vi "Visual Analyser.vi"(0 "Image In (RGB overlay)":T1, 1 "Buttons":T2, 2 "Indicators":T7, 3 "Dialog Indicator":refnum<vi>, 4 "Vision Frame":T1, 5 "Image Indicator":variant, 7 "Visualization Parameters":T3, 9 "Image Analysis":T6, 11 "Error In":errorcluster, 12 "Exploration and Autofocus":T4, 13 "Targeting Units":T5(array[cluster]), 14 "Transformation Matrix":refnum<vi>) -> (8 "Vision Frame Out":T1, 15 "Error Out":errorcluster)   [LabVIEW 2012, in "Visual Analyser.lvlib"]
uses:
  Visual Analyser.lvlib
  <vilib>/Analysis/Matrix/Datatypes/RealMatrix.ctl
  <vilib>/vision/Image Controls.llb/IMAQ Image.ctl
  <vilib>/vision/NI_Vision_Development_Module.lvlib
  <vilib>/Analysis/Matrix/NI_Matrix.lvlib
panel:
  out "Image Area":cluster{"X Resolution":i32, "Y Resolution":i32}
  out "Image":T1(plugin-control)
  out "Exit":bool
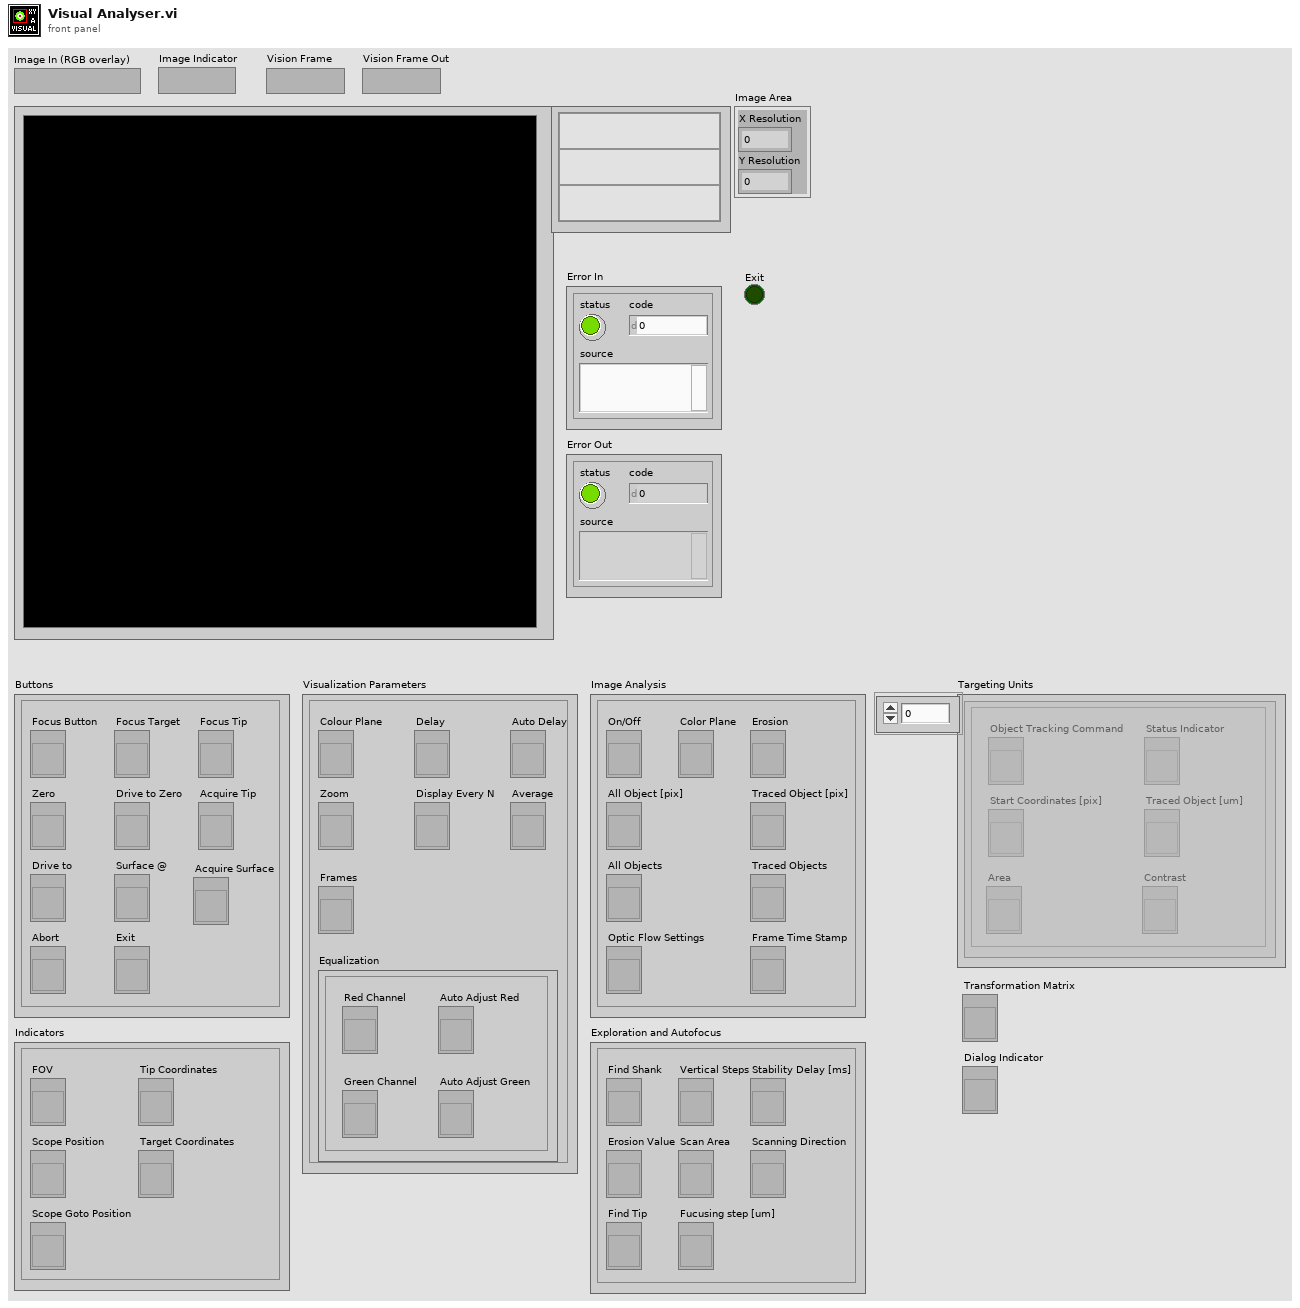
[diagram p1: front panel]
types:
  T1 = typedef "IMAQ Image.ctl" = refnum<image>
  T2 = cluster{"Focus Tip":refnum<vi>, "Focus Target":refnum<vi>, "Drive to Zero":refnum<vi>, "Zero":refnum<vi>, "Acquire Tip":refnum<vi>, "Focus Button":refnum<vi>, "Exit":refnum<vi>, "Abort":refnum<vi>, "Drive to":refnum<vi>, "Surface @":refnum<vi>, "Acquire Surface":refnum<vi>}
  T3 = cluster{"Display Every N":refnum<vi>, "Average":refnum<vi>, "Frames":refnum<vi>, "Colour Plane":refnum<vi>, "Zoom":refnum<vi>, "Delay":refnum<vi>, "Equalization":cluster{"Green Channel":refnum<vi>, "Auto Adjust Green":refnum<vi>, "Red Channel":refnum<vi>, "Auto Adjust Red":refnum<vi>}, "Auto Delay":refnum<vi>}
  T4 = cluster{"Find Shank":refnum<vi>, "Find Tip":refnum<vi>, "Scanning Direction":refnum<vi>, "Scan Area":refnum<vi>, "Stability Delay [ms]":refnum<vi>, "Vertical Steps":refnum<vi>, "Fucusing step [um]":refnum<vi>, "Erosion Value":refnum<vi>}
  T5 = cluster{"Object Tracking Command":refnum<vi>, "Status Indicator":refnum<vi>, "Start Coordinates [pix]":refnum<vi>, "Traced Object [um]":refnum<vi>, "Area":refnum<vi>, "Contrast":refnum<vi>}[]
  T6 = cluster{"On/Off":refnum<vi>, "All Objects":refnum<vi>, "Color Plane":refnum<vi>, "Erosion":refnum<vi>, "Traced Objects":refnum<vi>, "Frame Time Stamp":refnum<vi>, "Optic Flow Settings":refnum<vi>, "All Object [pix]":refnum<vi>, "Traced Object [pix]":refnum<vi>}
  T7 = cluster{"Tip Coordinates":refnum<vi>, "Target Coordinates":refnum<vi>, "Scope Position":refnum<vi>, "FOV":refnum<vi>, "Scope Goto Position":refnum<vi>}
  T8 = cluster{"Area":dbl, "Centre of Mass":cluster{"X":dbl, "Y":dbl}, "Global Rectangle":cluster{"Left":dbl, "Top":dbl, "Right":dbl, "Bottom":dbl}, "Contrast":dbl}[]
  T9 = cluster{"Pyramid Levels":i32, "Max Iterations":i32, "Displacement Threshold":dbl, "Window Size":i32}
  T10 = cluster{"X [um]":dbl, "Y [um]":dbl, "Z [um]":dbl}
  T11 = typedef "NI_Matrix.lvlib/RealMatrix.ctl" = dbl[][]
  T12 = cluster{"Erosion Value":refnum<vi>, "Fucusing step [um]":refnum<vi>, "Stability Delay [ms]":refnum<vi>}
  T13 = cluster{"Vertical Steps":refnum<vi>, "Stability Delay":refnum<vi>, "Scanning Direction":refnum<vi>, "Scan Area":refnum<vi>}
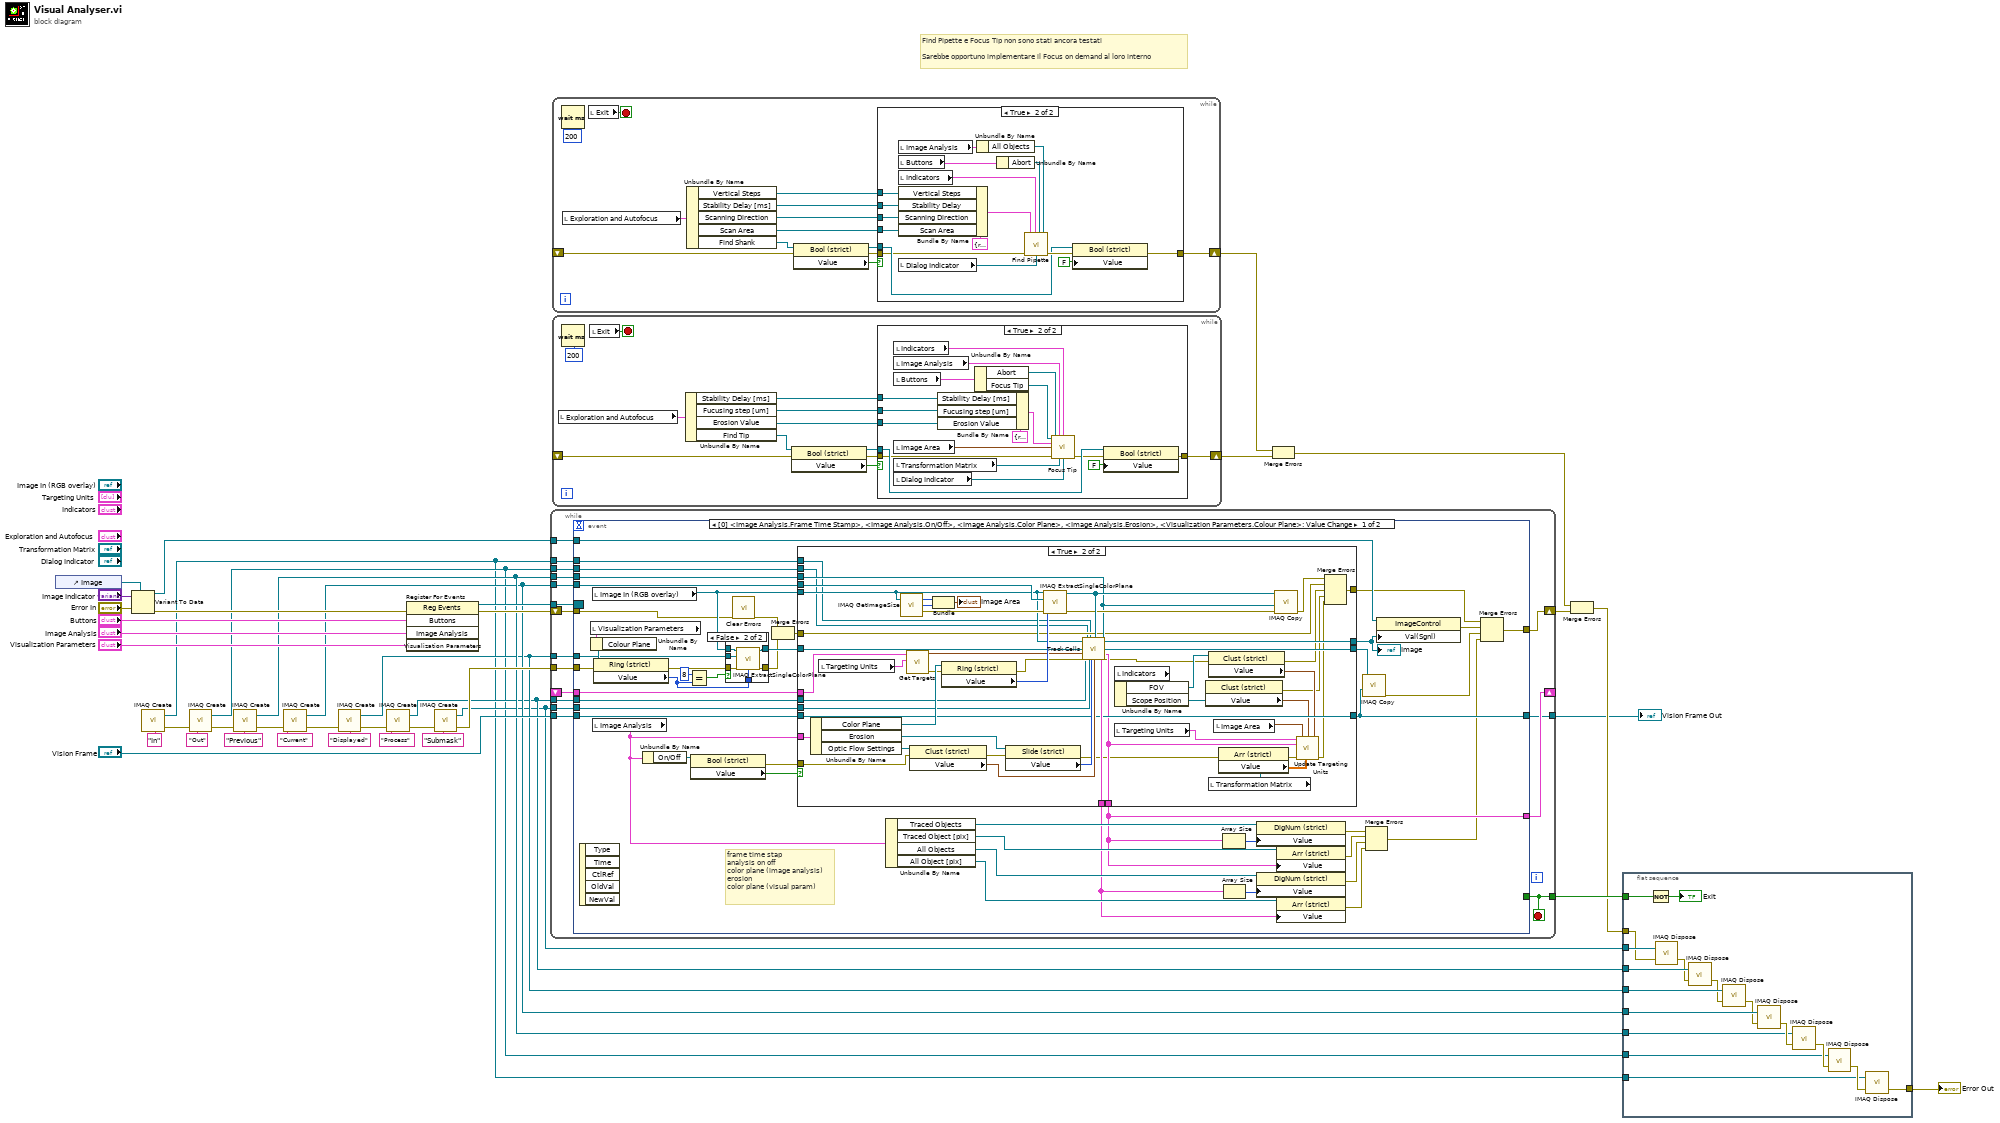
[diagram p0: block diagram]
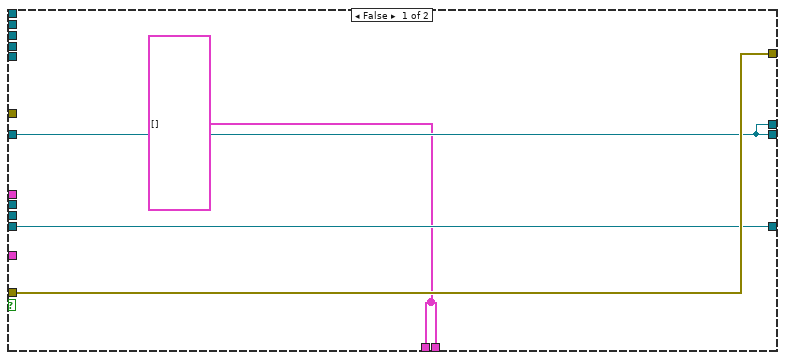
[diagram p5: hidden frame]
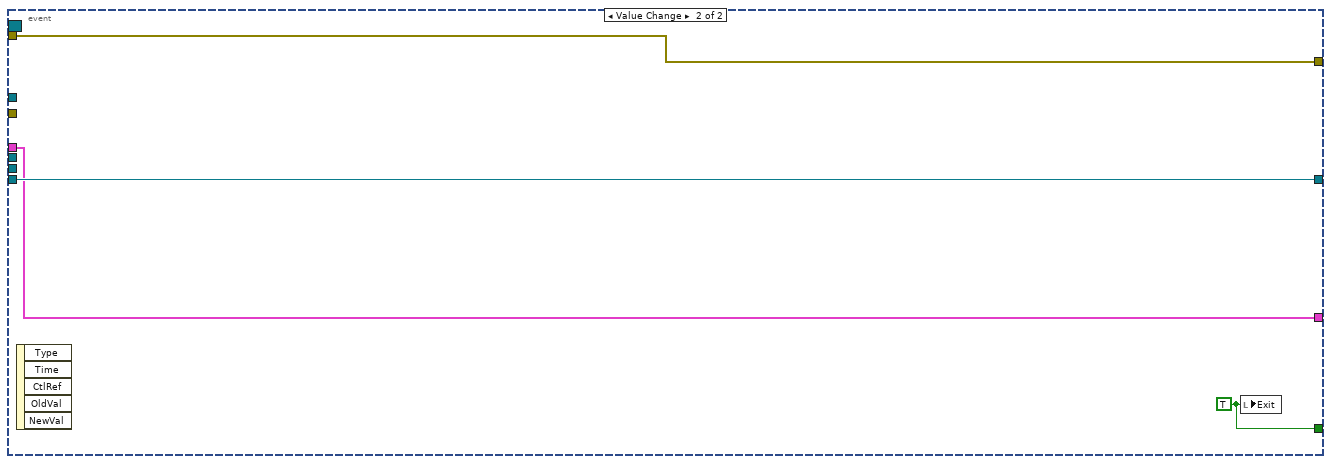
[diagram p6: hidden frame]
diagram:
  # "Find Pipette e Focus Tip non sono stati ancora testati\n\nSarebbe opportuno implementare il Focus on demand al loro interno"
  n1 = control-ref of="Image"() -> (w34:refnum<vi>)
  n2 = Variant To Data(error in="Error In", type=w34, Variant="Image Indicator") -> (data=w36:refnum<vi>, error out=w20:errorcluster)
  n3 = call "IMAQ Create"("Image Name"="In") -> ("New Image"=w1:T1, "error out"=w8:errorcluster)  [unwired: 4 in]
  n4 = call "IMAQ Create"("Image Name"="Out", "error in (no error)"=w8) -> ("New Image"=w2:T1, "error out"=w10:errorcluster)  [unwired: 3 in]
  n5 = call "IMAQ Create"("Image Name"="Previous", "error in (no error)"=w10) -> ("New Image"=w7:T1, "error out"=w32:errorcluster)  [unwired: 3 in]
  n6 = call "IMAQ Create"("Image Name"="Current", "error in (no error)"=w32) -> ("New Image"=w6:T1, "error out"=w24:errorcluster)  [unwired: 3 in]
  n7 = call "IMAQ Create"("Image Name"="Displayed", "error in (no error)"=w24) -> ("New Image"=w5:T1, "error out"=w33:errorcluster)  [unwired: 3 in]
  n8 = call "IMAQ Create"("Image Name"="Process", "error in (no error)"=w33) -> ("New Image"=w4:T1, "error out"=w13:errorcluster)  [unwired: 3 in]
  n9 = register-events(error in=w20, "Buttons", "Image Analysis", "Visualization Parameters") -> (reference out=w22:refnum<event-registration>, error out=w21:errorcluster)  [unwired: 1 in]
  n10 = call "IMAQ Create"("Image Name"="Submask", "error in (no error)"=w13) -> ("New Image"=w3:T1, "error out"=w12:errorcluster)  [unwired: 3 in]
  n11 = while {
    tunnel: w6 -> [w51]
    tunnel: w4 -> [w57]
    tunnel: w5 -> [w56]
    shift-right: [w54] -> _
    shift-left: _ -> [w55]
    tunnel: w36 -> [w49]
    tunnel: [w53] -> w31
    tunnel: w7 -> [w52]
    shift-right: [w47] -> w26
    shift-left: w21 -> [w48]
    tunnel: w12 -> [w50]
    tunnel: w22 -> [w46]
    tunnel: "Vision Frame" -> [w45]
    tunnel: [w44] -> w16
    tunnel: w3 -> [w43]
    tunnel: w2 -> [w42]
    tunnel: w1 -> [w41]
    stop <- w53 stop-if-true
    n12 = event shown="[0] <Image Analysis.Frame Time Stamp>, <Image Analysis.On/Off>, <Image Analysis.Color Plane>, <Image Analysis.Erosion>, <Visualization Parameters.Colour Plane>: Value Change" {
      selector: w46 -> [_ _]
      dyn-events: _ -> [_ _]
      timeout: _ -> [_ _]
      tunnel: w57 -> [w73 _]
      tunnel: w56 -> [w72 _]
      tunnel: w55 -> [w100 w168]
      tunnel: [w79 w168] -> w54
      tunnel: [_ w171] -> w53
      tunnel: w52 -> [w83 _]
      tunnel: w51 -> [w82 _]
      tunnel: w50 -> [w81 _]
      tunnel: w49 -> [w80 _]
      tunnel: w48 -> [w59 w170]
      tunnel: [w60 w170] -> w47
      tunnel: w45 -> [w70 w169]
      tunnel: [w69 w169] -> w44
      tunnel: w43 -> [w67 _]
      tunnel: w42 -> [w66 _]
      tunnel: w41 -> [w65 _]
      event Value Change {
        # "frame time stap\nanalysis on off\ncolor plane (image analysis)\nerosion\ncolor plane (visual param)"
        n13 = event-data() -> ()  [unwired: 1 in, 5 out]
        n14 = local read "Visualization Parameters"() -> (w84:T3)
        n15 = Unbundle By Name(w84) -> ("Colour Plane"=w92:refnum<vi>)
        n16 = local read "Image Analysis"() -> (w78:T6)
        n17 = local read "Image In (RGB overlay)"() -> (w77:T1)
        n18 = property on="Property Node" class="Ring (strict)"(reference=w92, error in=w81) -> (error out=w90:errorcluster, "Value"=w101:i32)  [unwired: 1 out]
        n19 = Unbundle By Name(w78) -> ("On/Off"=w93:refnum<vi>)
        n20 = Equal?(x=8, y=w101) -> (x = y?=w102:bool)
        n21 = property on="Property Node" class="Bool (strict)"(reference=w93) -> (error out=w91:errorcluster, "Value"=w104:bool)  [unwired: 1 in, 1 out]
        n22 = case shown="False" w102 {
          tunnel: w77 -> [w106 w112]
          tunnel: [w106 w111] -> w76
          tunnel: w72 -> [_ w110]
          tunnel: [w105 w109] -> w74
          tunnel: w101 -> [_ w108]
          tunnel: w90 -> [w105 w107]
          frame True {
          }
          frame False {
            n23 = call "IMAQ ExtractSingleColorPlane"("Color Plane"=w108, "error in (no error)"=w107, "Image Dst"=w110, "Image Src"=w112) -> ("error out"=w109:errorcluster, "Image Dst Out"=w111:T1)  [unwired: 6 in]
          }
        }
        n24 = call <vilib>:"Clear Errors.vi"("error in (no error)"=w59) -> ("error out"=w58:errorcluster)  [unwired: 6 in]
        n25 = Merge Errors(w58, w74) -> (w75:errorcluster)
        n26 = case shown="True" w104 {
          tunnel: w83 -> [_ w164]
          tunnel: w73 -> [_ w148]
          tunnel: w76 -> [w114 w149]
          tunnel: w82 -> [_ w155]
          tunnel: w100 -> [_ w143]
          tunnel: [w114 w146] -> w71
          tunnel: w77 -> [_ w125]
          tunnel: w91 -> [w116 w150]
          tunnel: w75 -> [_ w122]
          tunnel: [w116 w151] -> w64
          tunnel: [w113 w161] -> w89
          tunnel: [w113 w144] -> w79
          tunnel: w78 -> [_ w156]
          tunnel: w70 -> [w115 w147]
          tunnel: [w115 w147] -> w69
          tunnel: [w114 w145] -> w68
          tunnel: w67 -> [_ w121]
          tunnel: w66 -> [_ w119]
          tunnel: w65 -> [_ w120]
          frame False {
            w113 = T8 [] ("All Object [pix]")
          }
          frame True {
            n27 = Unbundle By Name(w156) -> ("Color Plane"=w163:refnum<vi>, "Erosion"=w159:refnum<vi>, "Optic Flow Settings"=w152:refnum<vi>)
            n28 = local read "Targeting Units"() -> (w142:T5)
            n29 = call "IMAQ GetImageSize"("Image"=w125) -> ("Y Resolution"=w128:i32, "X Resolution"=w129:i32, "error out"=w126:errorcluster)  [unwired: 1 in, 2 out]
            n30 = call "Get Targets.vi"("Targeting Units"=w142, "Target in [pix]"=w143) -> ("error out"=w153:errorcluster, "Objects to track Out [pix]"=w154:cluster{"X":dbl, "Y":dbl}[])  [unwired: 8 in]
            n31 = property on="Property Node" class="Clust (strict)"(reference=w152, error in=w150) -> (error out=w160:errorcluster, "Value"=w157:T9)  [unwired: 1 out]
            n32 = Bundle("X Resolution"=w129, "Y Resolution"=w128) -> (→"Image Area":cluster{"X Resolution":i32, "Y Resolution":i32})  [unwired: 1 out]
            n33 = property on="Property Node" class="Ring (strict)"(reference=w163, error in=w153) -> (error out=w162:errorcluster, "Value"=w167:i32)  [unwired: 1 out]
            n34 = property on="Property Node" class="Slide (strict)"(reference=w159, error in=w160) -> (error out=w117:errorcluster, "Value"=w158:u32)  [unwired: 1 out]
            n35 = call "IMAQ ExtractSingleColorPlane"("Color Plane"=w167, "error in (no error)"=w126, "Image Dst"=w155, "Image Src"=w125) -> ("error out"=w165:errorcluster, "Image Dst Out"=w166:T1)  [unwired: 6 in]
            n36 = call "Track Cells.vi"("Previous Image In"=w164, "Current Image In"=w166, "Process Image In"=w148, "Overlapped Image"=w149, "Objects to track In [pix]"=w154, "RGB in"=w125, "error in"=w162, "In"=w119, "Optic Flow Settings"=w157, "Out"=w120, "Submask"=w121, "Erosion"=w158) -> ("Overlapped Image Out"=w146:T1, "All Object [pix]"=w161:T8, "Traced Object [pix]"=w144:T8, "RGB out"=w145:T1, "error out"=w118:errorcluster)  [unwired: 9 in, 2 out]
            n37 = local read "Targeting Units"() -> (w132:T5)
            n38 = local read "Indicators"() -> (w138:T7)
            n39 = Unbundle By Name(w138) -> ("FOV"=w135:refnum<vi>, "Scope Position"=w137:refnum<vi>)
            n40 = property class="Clust (strict)"(reference=w137) -> (error out=w130:errorcluster, "Value"=w136:T10)  [unwired: 1 in, 1 out]
            n41 = property class="Clust (strict)"(reference=w135, error in=w118) -> (error out=w134:errorcluster, "Value"=w133:cluster{"FOVx [um]":dbl, "FOVy [um]":dbl})  [unwired: 1 out]
            n42 = local read "Transformation Matrix"() -> (w141:refnum<vi>)
            n43 = local read "Image Area"() -> (w124:cluster{"X Resolution":i32, "Y Resolution":i32})
            n44 = property on="Property Node" class="Arr (strict)"(reference=w141, error in=w117) -> (error out=w139:errorcluster, "Value"=w140:T11)  [unwired: 1 out]
            n45 = call "IMAQ Copy"("error in (no error)"=w165, "Image Dst"=w164, "Image Src"=w166) -> ("error out"=w123:errorcluster)  [unwired: 4 out]
            n46 = call "Update Targeting Units.vi"("Targeting Units"=w132, "Scope Position"=w136, "Object In [pix]"=w144, "error in (no error)"=w139, "FOV"=w133, "Image Area"=w124, "Transformation Matrix"=w140) -> ("error out"=w131:errorcluster)  [unwired: 7 in, 1 out]
            n47 = Merge Errors(w123, w122, w134, w130, w131) -> (w151:errorcluster)
          }
        }
        "Image" <- w71
        n48 = Unbundle By Name(w78) -> ("Traced Objects"=w98:refnum<vi>, "Traced Object [pix]"=w99:refnum<vi>, "All Objects"=w97:refnum<vi>, "All Object [pix]"=w96:refnum<vi>)
        n49 = Array Size(array=w79) -> (size(s)=w95:i32)
        n50 = Array Size(array=w89) -> (size(s)=w94:i32)
        n51 = property on="Property Node" class="DigNum (strict)"(reference=w98, "Value"=w95) -> (error out=w88:errorcluster)  [unwired: 1 in, 1 out]
        n52 = property on="Property Node" class="DigNum (strict)"(reference=w97, "Value"=w94) -> (error out=w86:errorcluster)  [unwired: 1 in, 1 out]
        n53 = property on="Property Node" class="Arr (strict)"(reference=w99, "Value"=w79) -> (error out=w87:errorcluster)  [unwired: 1 in, 1 out]
        n54 = property on="Property Node" class="Arr (strict)"(reference=w96, "Value"=w89) -> (error out=w85:errorcluster)  [unwired: 1 in, 1 out]
        n55 = call "IMAQ Copy"("Image Dst"=w69, "Image Src"=w68) -> ("error out"=w62:errorcluster)  [unwired: 1 in, 4 out]
        n56 = Merge Errors(w88, w87, w86, w85) -> (w61:errorcluster)
        n57 = property class="ImageControl"(reference=w80, "Val(Sgnl)"=w71) -> (error out=w63:errorcluster)  [unwired: 1 in, 1 out]
        n58 = Merge Errors(w64, w63, w62, w61) -> (w60:errorcluster)
      }
      event Value Change {
        w171 = TRUE ("Exit")
        n59 = event-data() -> ()  [unwired: 1 in, 5 out]
        n60 = local write "Exit"(w171) -> ()
      }
    }
  }
  "Vision Frame Out" <- w16
  n61 = while {
    shift-right: [w180] -> w28
    shift-left: _ -> [w178]
    stop <- w183 stop-if-true
    n62 = local read "Exploration and Autofocus"() -> (w175:T4)
    n63 = Wait (ms)(milliseconds to wait=u32 200) -> ()  [unwired: 1 out]
    n64 = local read "Exit"() -> (w183:bool)
    n65 = Unbundle By Name(w175) -> ("Stability Delay [ms]"=w174:refnum<vi>, "Fucusing step [um]"=w173:refnum<vi>, "Erosion Value"=w172:refnum<vi>, "Find Tip"=w176:refnum<vi>)
    n66 = property class="Bool (strict)"(reference=w176, error in=w178) -> (reference out=w179:refnum<vi>, error out=w181:errorcluster, "Value"=w182:bool)
    n67 = case shown="True" w182 {
      tunnel: w181 -> [w184 w200]
      tunnel: [w184 w202] -> w180
      tunnel: w179 -> [_ w201]
      tunnel: w174 -> [_ w195]
      tunnel: w173 -> [_ w194]
      tunnel: w172 -> [_ w193]
      frame False {
      }
      frame True {
        n68 = local read "Indicators"() -> (w190:T7)
        n69 = local read "Image Analysis"() -> (w185:T6)
        n70 = local read "Buttons"() -> (w189:T2)
        n71 = local read "Image Area"() -> (w191:cluster{"X Resolution":i32, "Y Resolution":i32})
        n72 = local read "Transformation Matrix"() -> (w186:refnum<vi>)
        n73 = local read "Dialog Indicator"() -> (w198:refnum<vi>)
        n74 = Bundle By Name(cluster=T12 {"Erosion Value"=refnum, "Fucusing step [um]"=refnum, "Stability Delay [ms]"=refnum} ("Focusing Parameters"), "Stability Delay [ms]"=w195, "Fucusing step [um]"=w194, "Erosion Value"=w193) -> (w192:T12)
        n75 = Unbundle By Name(w189) -> ("Abort"=w187:refnum<vi>, "Focus Tip"=w188:refnum<vi>)
        n76 = call "Focus Tip.vi"("Focus Tip"=w188, "Image Analysis"=w185, "Indicators"=w190, "Focusing Parameters"=w192, "Image Area"=w191, "error in (no error)"=w200, "Transformation Matrix"=w186, "Indicator"=w198, "Abort"=w187) -> ("error out"=w197:errorcluster)  [unwired: 6 in]
        n77 = property class="Bool (strict)"(reference=w201, error in=w197, "Value"=FALSE) -> (error out=w202:errorcluster)  [unwired: 1 out]
      }
    }
  }
  n78 = while {
    shift-right: [w212] -> w29
    shift-left: _ -> [w210]
    stop <- w215 stop-if-true
    n79 = Wait (ms)(milliseconds to wait=u32 200) -> ()  [unwired: 1 out]
    n80 = local read "Exploration and Autofocus"() -> (w207:T4)
    n81 = local read "Exit"() -> (w215:bool)
    n82 = Unbundle By Name(w207) -> ("Vertical Steps"=w203:refnum<vi>, "Stability Delay [ms]"=w204:refnum<vi>, "Scanning Direction"=w205:refnum<vi>, "Scan Area"=w206:refnum<vi>, "Find Shank"=w209:refnum<vi>)
    n83 = property class="Bool (strict)"(reference=w209, error in=w210) -> (reference out=w211:refnum<vi>, error out=w213:errorcluster, "Value"=w214:bool)
    n84 = case shown="True" w214 {
      tunnel: w213 -> [w216 w226]
      tunnel: [w216 w231] -> w212
      tunnel: w211 -> [_ w230]
      tunnel: w206 -> [_ w221]
      tunnel: w205 -> [_ w220]
      tunnel: w204 -> [_ w219]
      tunnel: w203 -> [_ w218]
      frame False {
      }
      frame True {
        n85 = local read "Image Analysis"() -> (w232:T6)
        n86 = local read "Buttons"() -> (w228:T2)
        n87 = local read "Indicators"() -> (w223:T7)
        n88 = Bundle By Name(cluster=T13 {"Vertical Steps"=refnum, "Stability Delay"=refnum, "Scanning Direction"=refnum, "Scan Area"=refnum} ("Scanning Parameters"), "Vertical Steps"=w218, "Stability Delay"=w219, "Scanning Direction"=w220, "Scan Area"=w221) -> (w217:T13)
        n89 = local read "Dialog Indicator"() -> (w225:refnum<vi>)
        n90 = Unbundle By Name(w232) -> ("All Objects"=w224:refnum<vi>)
        n91 = Unbundle By Name(w228) -> ("Abort"=w227:refnum<vi>)
        n92 = call "Find Pipette.vi"("Scanning Parameters"=w217, "Indicators"=w223, "Objects"=w224, "error in (no error)"=w226, "Indicator"=w225, "Abort ref"=w227) -> ("error out"=w233:errorcluster)  [unwired: 8 in, 1 out]
        n93 = property class="Bool (strict)"(reference=w230, error in=w233, "Value"=FALSE) -> (error out=w231:errorcluster)  [unwired: 1 out]
      }
    }
  }
  n94 = Merge Errors(w29, w28) -> (w25:errorcluster)
  n95 = Merge Errors(w25, w26) -> (w27:errorcluster)
  n96 = flat-sequence {
    tunnel: w3 -> [w250]
    tunnel: w4 -> [w249]
    tunnel: w5 -> [w248]
    tunnel: w6 -> [w247]
    tunnel: w27 -> [w243]
    tunnel: w31 -> [w241]
    tunnel: [w234] -> w30
    tunnel: w7 -> [w237]
    tunnel: w2 -> [w236]
    tunnel: w1 -> [w235]
    frame #0 {
      n97 = Not(x=w241) -> (.not. x?=→"Exit":bool)
      n98 = call "IMAQ Dispose"("Image"=w250, "error in (no error)"=w243) -> ("error out"=w246:errorcluster)  [unwired: 4 in]
      n99 = call "IMAQ Dispose"("Image"=w249, "error in (no error)"=w246) -> ("error out"=w245:errorcluster)  [unwired: 4 in]
      n100 = call "IMAQ Dispose"("Image"=w248, "error in (no error)"=w245) -> ("error out"=w244:errorcluster)  [unwired: 4 in]
      n101 = call "IMAQ Dispose"("Image"=w247, "error in (no error)"=w244) -> ("error out"=w240:errorcluster)  [unwired: 4 in]
      n102 = call "IMAQ Dispose"("Image"=w237, "error in (no error)"=w240) -> ("error out"=w239:errorcluster)  [unwired: 4 in]
      n103 = call "IMAQ Dispose"("Image"=w236, "error in (no error)"=w239) -> ("error out"=w238:errorcluster)  [unwired: 4 in]
      n104 = call "IMAQ Dispose"("Image"=w235, "error in (no error)"=w238) -> ("error out"=w234:errorcluster)  [unwired: 4 in]
    }
  }
  "Error Out" <- w30
